vi "Query Position and Record.vi"(8 "error in (no error)":errorcluster, 10 "SelectKey(True)":bool, 11 "ListSelection in":refnum<class "ListSelection.lvclass">) -> (0 "error out":errorcluster, 1 "SignedResult(\"\")":string, 2 "InxOfColumns":i32, 3 "ListSelection out":refnum<class "ListSelection.lvclass">)   [LabVIEW 2015, in "Admin_Actor.lvlib" / "ListSelection.lvclass"]
uses:
  ListSelection.lvclass
  ListSelection.lvclass/ListSelection.ctl
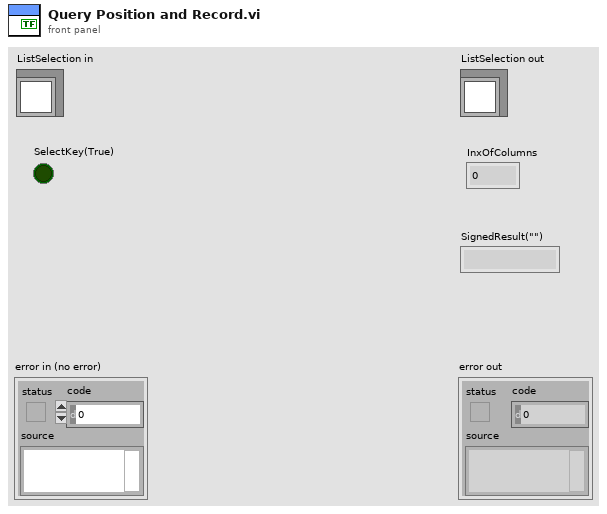
[diagram p1: front panel]
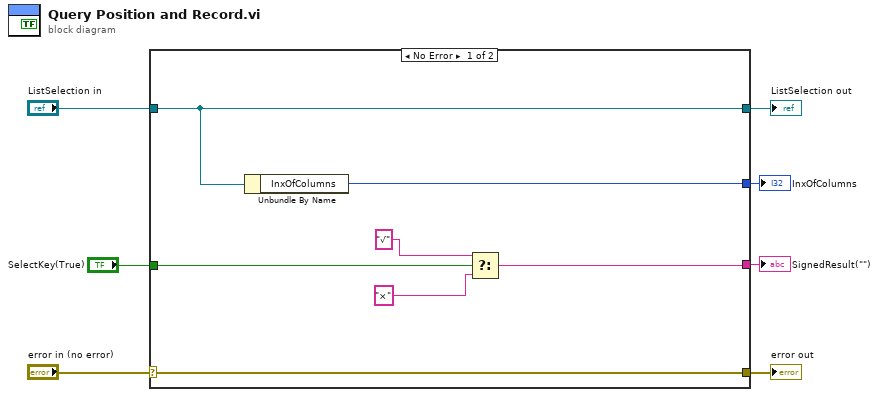
[diagram p0: block diagram]
diagram:
  n1 = case shown="No Error" "error in (no error)" {
    selector: "error in (no error)" -> [w14 w16]
    tunnel: [w14 w16] -> w6
    tunnel: [w13 w15] -> w4
    tunnel: "ListSelection in" -> [w13 w15]
    tunnel: [w12 _] -> w3
    tunnel: "SelectKey(True)" -> [w11 _]
    tunnel: [w8 _] -> w1
    frame No Error {
      n2 = Unbundle By Name(w13) -> ("InxOfColumns"=w12:i32)
      n3 = Select(t="√", s=w11, f="×") -> (s? t:f=w8:string)
    }
    frame Error {
    }
  }
  "error out" <- w6
  "ListSelection out" <- w4
  "InxOfColumns" <- w3
  "SignedResult(\"\")" <- w1
